vi "智能交通灯.vi"() -> ()   [LabVIEW 2024]
uses:
  <vilib>/Utility/file.llb/Read From Spreadsheet File (DBL).vi
panel:
  in  "?":u16(ring) items=["无", "黄灯常亮", "南北通行", "东西通行"]
  in  "手动\n\n自动":bool
  in  "道路宽度":dbl
  in  "人流量":dbl
  in  "车流量":dbl
  in  "模式切换":bool
  out "日志":string
  out "自动模式":bool
  in  "绿灯时间":i32
  in  "红灯时间":i32
  in  "黄灯时间":i32
  out "手动模式":bool
  out "北红":bool
  out "北绿":bool
  out "北黄":bool
  out "北灯":dbl
  out "南黄":bool
  out "南红":bool
  out "南绿":bool
  out "南灯":dbl
  out "西绿":bool
  out "西黄":bool
  out "西红":bool
  out "西灯":dbl
  out "东黄":bool
  out "东绿":bool
  out "东红":bool
  out "东灯":dbl
  # "交通灯控制交互界面"
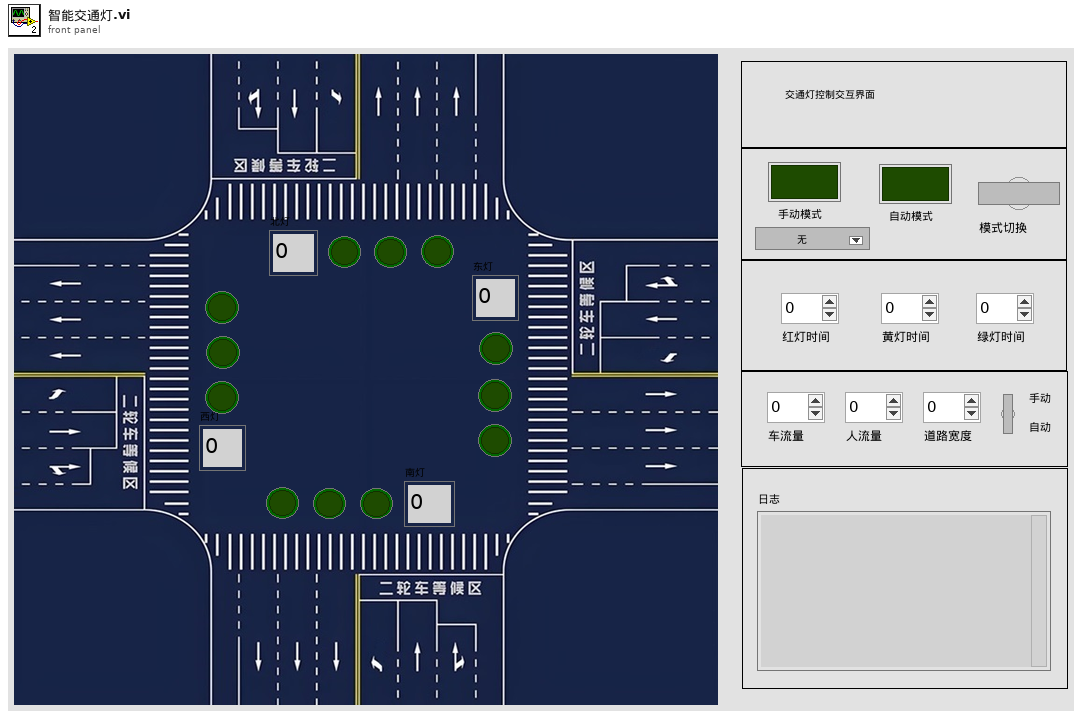
[diagram p1: front panel]
types:
  T1 = cluster{"first row[0]":dbl, "first row[1]":dbl, "first row[2]":dbl}
  T2 = cluster{"[0]":bool, "[1]":bool, "[2]":bool, "[3]":bool, "[4]":bool, "[5]":bool, "[6]":bool, "[7]":bool, "[8]":bool, "[9]":bool, "[10]":bool, "[11]":bool}
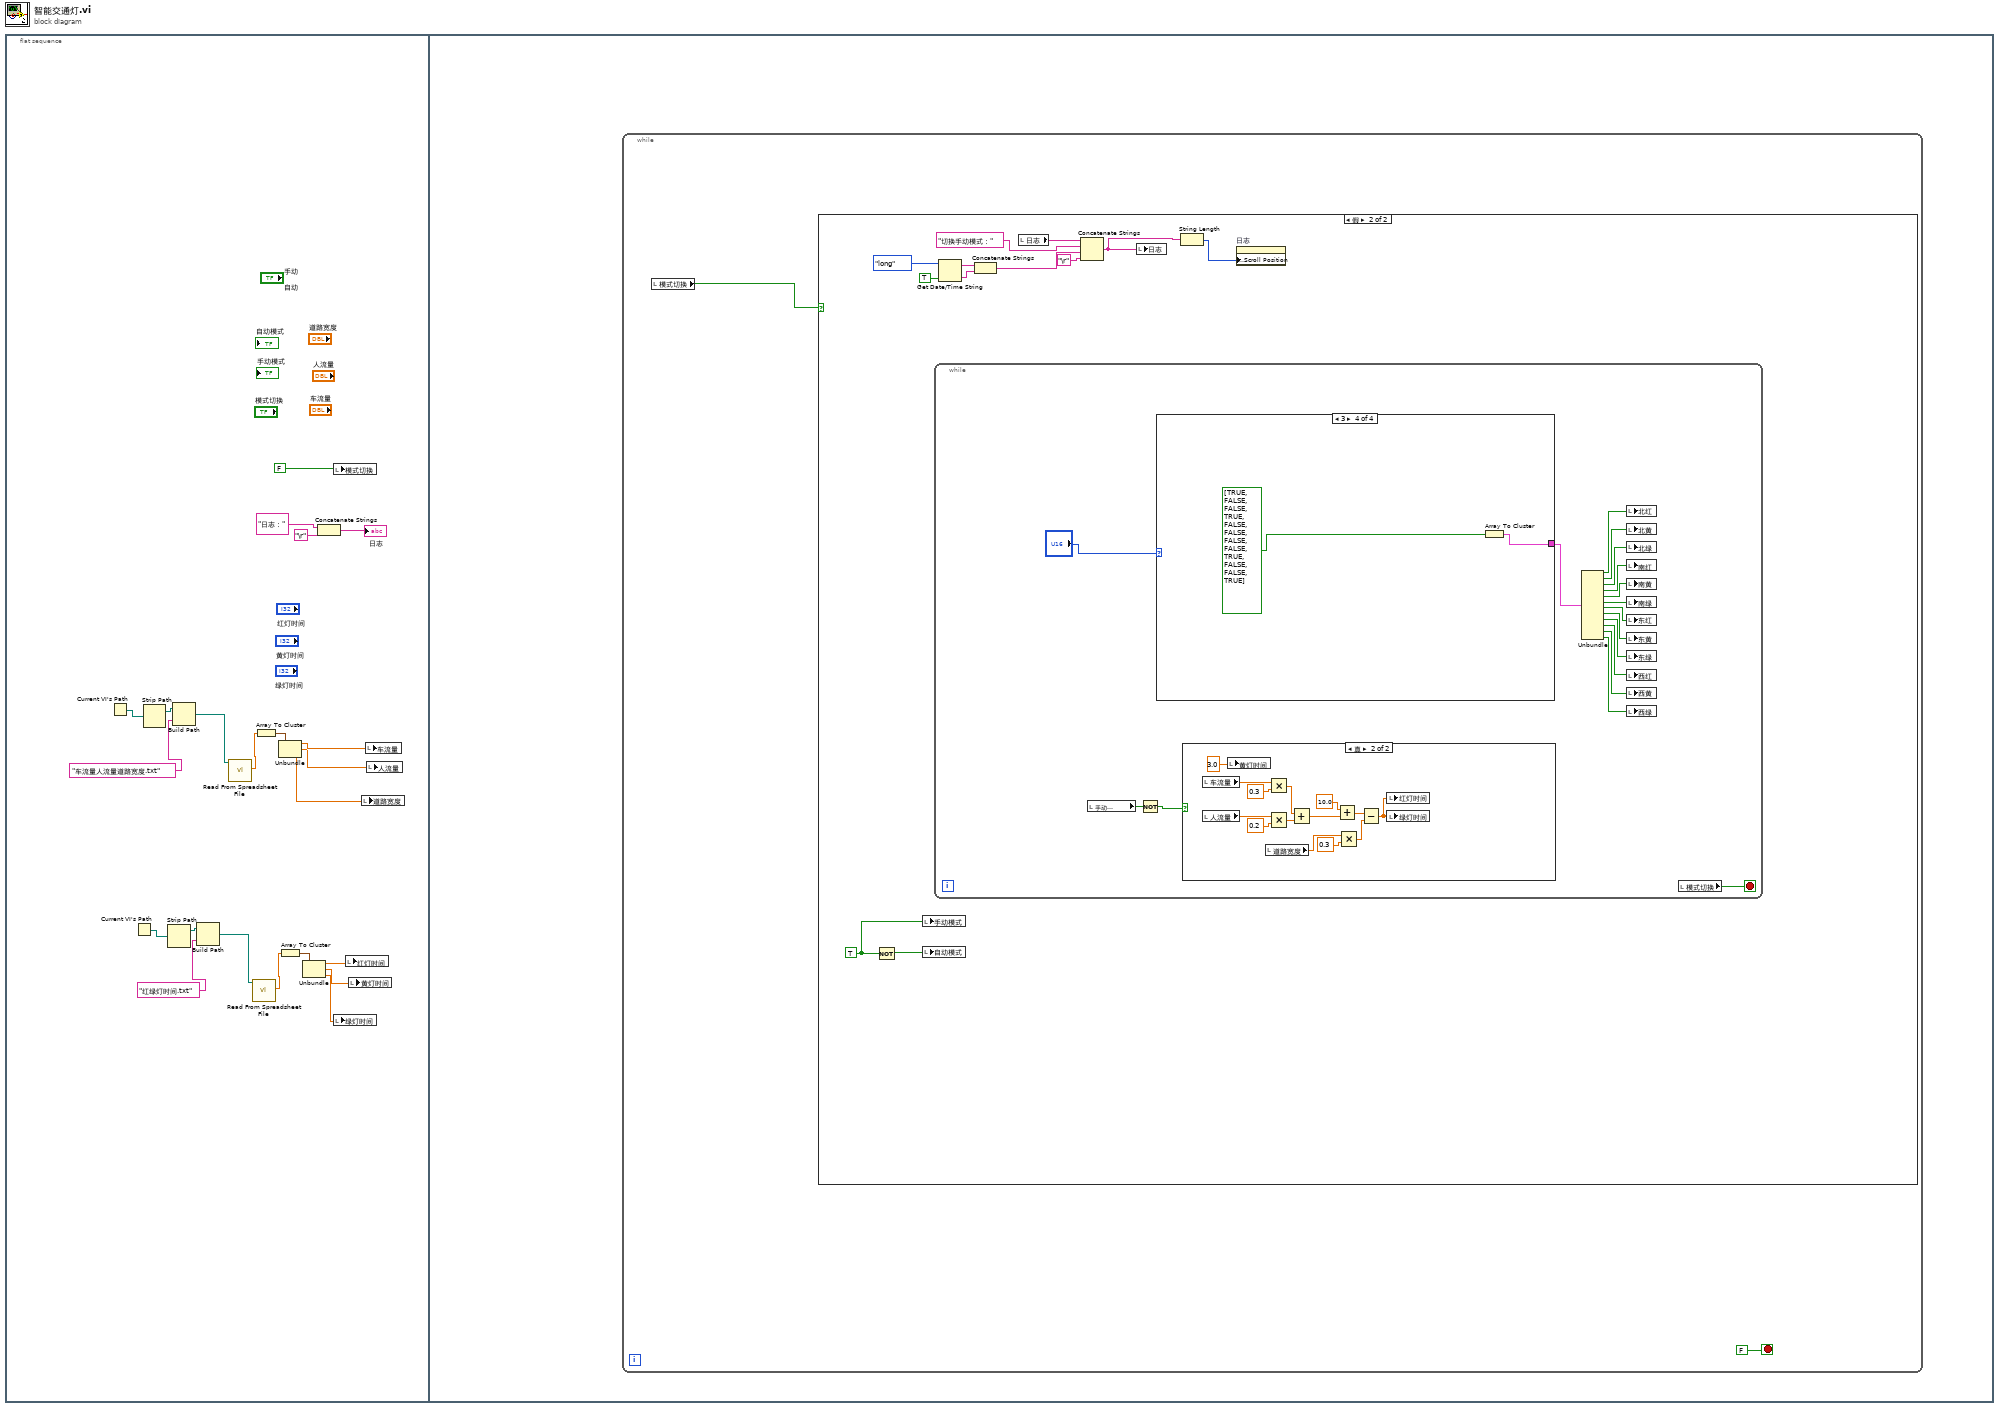
[diagram p0: block diagram]
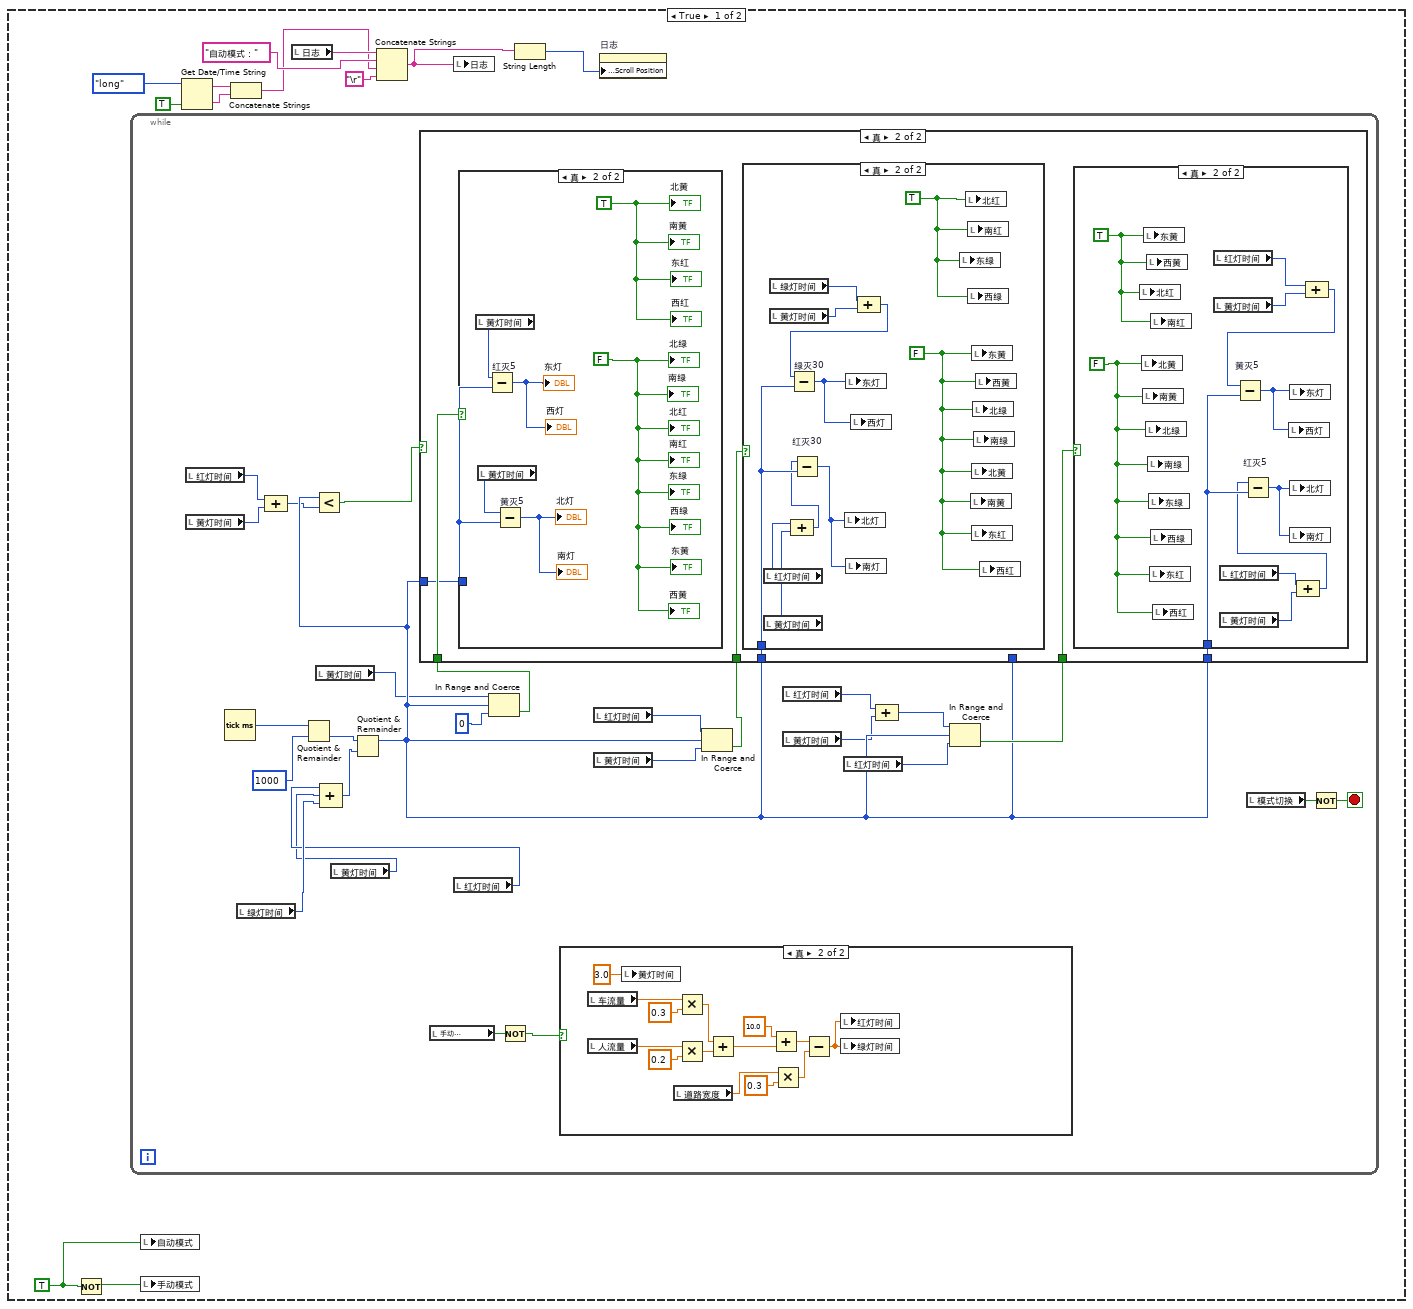
[diagram p2: hidden frame]
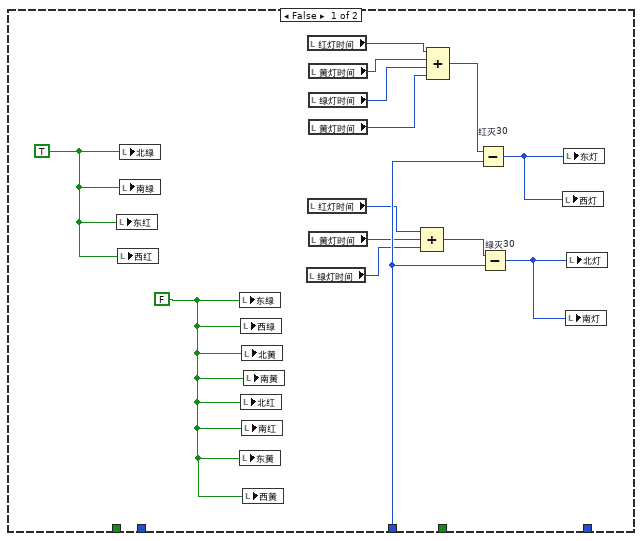
[diagram p4: hidden frame]
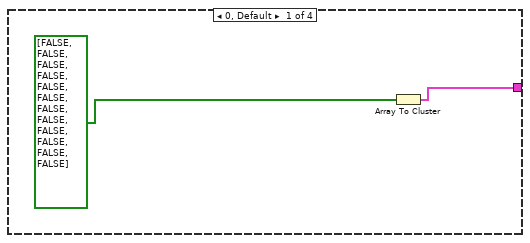
[diagram p8: hidden frame]
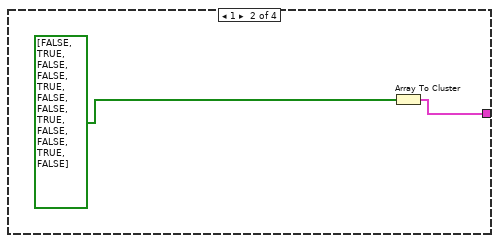
[diagram p9: hidden frame]
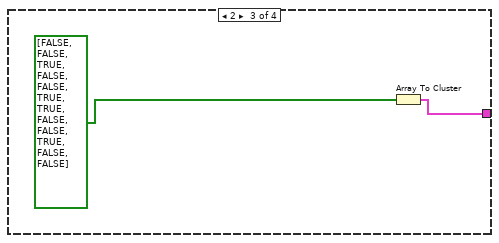
[diagram p10: hidden frame]
diagram:
  n1 = flat-sequence {
    frame #0 {
      n2 = Current VI's Path() -> (path=w4:path)
      n3 = Current VI's Path() -> (path=w18:path)
      n4 = Strip Path(path=w4) -> (stripped path=w5:path)  [unwired: 1 out]
      n5 = Strip Path(path=w18) -> (stripped path=w17:path)  [unwired: 1 out]
      n6 = Build Path(base path=w5, name or relative path="车流量人流量道路宽度.txt" ("名称")) -> (appended path=w7:path)
      n7 = Build Path(base path=w17, name or relative path="红绿灯时间.txt" ("名称")) -> (appended path=w15:path)
      n8 = call-poly <vilib>:"Read From Spreadsheet File.vi"("file path (dialog if empty)"=w7) -> ("first row"=w8:dbl[])  [unwired: 6 in, 4 out]
      n9 = call-poly <vilib>:"Read From Spreadsheet File.vi"("file path (dialog if empty)"=w15) -> ("first row"=w14:dbl[])  [unwired: 6 in, 4 out]
      n10 = Array To Cluster(array=w8) -> (cluster=w9:T1)
      n11 = Unbundle(w9) -> ("first row[0]"=w3:dbl, "first row[1]"=w2:dbl, "first row[2]"=w1:dbl)
      n12 = Array To Cluster(array=w14) -> (cluster=w13:T1)
      n13 = Unbundle(w13) -> ("first row[0]"=w12:dbl, "first row[1]"=w11:dbl, "first row[2]"=w10:dbl)
      n14 = Concatenate Strings("日志：" ("日志"), "\r") -> (→"日志":string)
      n15 = local write "模式切换"(FALSE) -> ()
      n16 = local write "绿灯时间"(w10) -> ()
      n17 = local write "红灯时间"(w12) -> ()
      n18 = local write "黄灯时间"(w11) -> ()
      n19 = local write "道路宽度"(w1) -> ()
      n20 = local write "车流量"(w3) -> ()
      n21 = local write "人流量"(w2) -> ()
    }
    frame #1 {
      n22 = while {
        stop <- FALSE stop-if-true
        n23 = local read "模式切换"() -> (w23:bool)
        n24 = case shown="假" w23 {
          frame True {
            w35 = TRUE
            n25 = Not(x=w35) -> (.not. x?=w36:bool)
            n26 = while {
              stop <- w40 stop-if-true
              n27 = local read "红灯时间"() -> (w51:i32)
              n28 = local read "黄灯时间"() -> (w50:i32)
              n29 = Tick Count (ms)() -> (millisecond timer value=w63:u32)
              n30 = local read "绿灯时间"() -> (w43:i32)
              n31 = Compound Arithmetic op=ADD(w51, w50) -> (w53:i32)
              n32 = Quotient & Remainder(x=w63, y=1000) -> (floor(x/y)=w60:u32)  [unwired: 1 out]
              n33 = local read "黄灯时间"() -> (w49:i32)
              n34 = local read "黄灯时间"() -> (w41:i32)
              n35 = local read "手动\n\n自动"() -> (w38:bool)
              n36 = local read "红灯时间"() -> (w42:i32)
              n37 = Compound Arithmetic op=ADD(w42, w41, w43) -> (w54:i32)
              n38 = Quotient & Remainder(x=w60, y=w54) -> (x-y*floor(x/y)=w55:u32)  [unwired: 1 out]
              n39 = Less?(x=w55, y=w53) -> (x < y?=w59:bool)
              n40 = In Range and Coerce(upper limit=w49, x=w55, lower limit=0) -> (In Range?=w58:bool)  [unwired: 1 out]
              n41 = Not(x=w38) -> (.not. x?=w37:bool)
              n42 = case shown="真" w37 {
                frame False {
                }
                frame True {
                  n43 = local read "车流量"() -> (w77:dbl)
                  n44 = local read "人流量"() -> (w75:dbl)
                  n45 = local write "黄灯时间"(3.0 ("黄灯时间")) -> ()
                  n46 = local read "道路宽度"() -> (w68:dbl)
                  n47 = Multiply(x=w77, y=0.3) -> (x*y=w73:dbl)
                  n48 = Multiply(x=w75, y=0.2) -> (x*y=w72:dbl)
                  n49 = Add(x=w73, y=w72) -> (x+y=w70:dbl)
                  n50 = Add(x=10.0, y=w70) -> (x+y=w69:dbl)
                  n51 = Multiply(x=w68, y=0.3) -> (x*y=w66:dbl)
                  n52 = Subtract(x=w69, y=w66) -> (x-y=w65:dbl)
                  n53 = local write "红灯时间"(w65) -> ()
                  n54 = local write "绿灯时间"(w65) -> ()
                }
              }
              n55 = local read "红灯时间"() -> (w48:i32)
              n56 = local read "黄灯时间"() -> (w47:i32)
              n57 = In Range and Coerce(upper limit=w48, x=w55, lower limit=w47) -> (In Range?=w57:bool)  [unwired: 1 out]
              n58 = local read "红灯时间"() -> (w46:i32)
              n59 = local read "黄灯时间"() -> (w45:i32)
              n60 = local read "红灯时间"() -> (w44:i32)
              n61 = Compound Arithmetic op=ADD(w46, w45) -> (w52:i32)
              n62 = In Range and Coerce(upper limit=w52, x=w55, lower limit=w44) -> (In Range?=w56:bool)  [unwired: 1 out]
              n63 = case shown="真" w59 {
                tunnel: w58 -> [_ w97]
                tunnel: w55 -> [_ w96]
                tunnel: w55 -> [_ w95]
                tunnel: w55 -> [_ w94]
                tunnel: w57 -> [_ w93]
                tunnel: w56 -> [_ w92]
                tunnel: w55 -> [w91 _]
                frame False {
                  w87 = FALSE
                  w88 = TRUE
                  n64 = local write "东红"(w88) -> ()
                  n65 = local write "西红"(w88) -> ()
                  n66 = local write "北绿"(w88) -> ()
                  n67 = local write "南绿"(w88) -> ()
                  n68 = local write "东绿"(w87) -> ()
                  n69 = local write "东黄"(w87) -> ()
                  n70 = local write "西绿"(w87) -> ()
                  n71 = local write "北红"(w87) -> ()
                  n72 = local write "北黄"(w87) -> ()
                  n73 = local write "南红"(w87) -> ()
                  n74 = local write "西黄"(w87) -> ()
                  n75 = local write "南黄"(w87) -> ()
                  n76 = local read "绿灯时间"() -> (w83:i32)
                  n77 = local read "红灯时间"() -> (w81:i32)
                  n78 = local read "红灯时间"() -> (w84:i32)
                  n79 = local read "黄灯时间"() -> (w80:i32)
                  n80 = local read "绿灯时间"() -> (w79:i32)
                  n81 = local read "黄灯时间"() -> (w78:i32)
                  n82 = local read "黄灯时间"() -> (w82:i32)
                  n83 = Compound Arithmetic op=ADD(w84, w82, w83) -> (w86:i32)
                  n84 = Compound Arithmetic op=ADD(w81, w80, w79, w78) -> (w85:i32)
                  n85 = Subtract "红灭30"(x=w85, y=w91) -> (x-y=w90:u32)
                  n86 = Subtract "绿灭30"(x=w86, y=w91) -> (x-y=w89:u32)
                  n87 = local write "西灯"(w90) -> ()
                  n88 = local write "东灯"(w90) -> ()
                  n89 = local write "南灯"(w89) -> ()
                  n90 = local write "北灯"(w89) -> ()
                }
                frame True {
                  n91 = case shown="真" w97 {
                    tunnel: w96 -> [_ w104]
                    frame False {
                    }
                    frame True {
                      w100 = FALSE
                      w103 = TRUE ("布尔")
                      n92 = local read "黄灯时间"() -> (w99:i32)
                      n93 = local read "黄灯时间"() -> (w98:i32)
                      n94 = Subtract "红灭5"(x=w99, y=w104) -> (x-y=→"东灯" →"西灯":u32)
                      n95 = Subtract "黄灭5"(x=w98, y=w104) -> (x-y=→"北灯" →"南灯":u32)
                      "北黄" <- w103
                      "北绿" <- w100
                      "东红" <- w103
                      "东黄" <- w100
                      "北红" <- w100
                      "东绿" <- w100
                      "南黄" <- w103
                      "西红" <- w103
                      "南绿" <- w100
                      "南红" <- w100
                      "西绿" <- w100
                      "西黄" <- w100
                    }
                  }
                  n96 = case shown="真" w93 {
                    tunnel: w94 -> [_ w126]
                    frame False {
                    }
                    frame True {
                      w122 = FALSE
                      w125 = TRUE
                      n97 = local read "红灯时间"() -> (w120:i32)
                      n98 = local read "黄灯时间"() -> (w119:i32)
                      n99 = local read "绿灯时间"() -> (w118:i32)
                      n100 = local read "黄灯时间"() -> (w117:i32)
                      n101 = Compound Arithmetic op=ADD(w120, w119) -> (w121:i32)
                      n102 = Subtract "红灭30"(x=w121, y=w126) -> (x-y=w123:u32)
                      n103 = local write "北灯"(w123) -> ()
                      n104 = local write "南灯"(w123) -> ()
                      n105 = Compound Arithmetic op=ADD(w118, w117) -> (w116:i32)
                      n106 = Subtract "绿灭30"(x=w116, y=w126) -> (x-y=w124:u32)
                      n107 = local write "东灯"(w124) -> ()
                      n108 = local write "西灯"(w124) -> ()
                      n109 = local write "东绿"(w125) -> ()
                      n110 = local write "北红"(w125) -> ()
                      n111 = local write "南红"(w125) -> ()
                      n112 = local write "西绿"(w125) -> ()
                      n113 = local write "南黄"(w122) -> ()
                      n114 = local write "东黄"(w122) -> ()
                      n115 = local write "北黄"(w122) -> ()
                      n116 = local write "东红"(w122) -> ()
                      n117 = local write "北绿"(w122) -> ()
                      n118 = local write "南绿"(w122) -> ()
                      n119 = local write "西黄"(w122) -> ()
                      n120 = local write "西红"(w122) -> ()
                    }
                  }
                  n121 = case shown="真" w92 {
                    tunnel: w95 -> [_ w115]
                    frame False {
                    }
                    frame True {
                      w113 = FALSE
                      w114 = TRUE
                      n122 = local write "北红"(w114) -> ()
                      n123 = local write "北黄"(w113) -> ()
                      n124 = local write "南黄"(w113) -> ()
                      n125 = local write "东黄"(w114) -> ()
                      n126 = local write "北绿"(w113) -> ()
                      n127 = local write "西黄"(w114) -> ()
                      n128 = local write "南绿"(w113) -> ()
                      n129 = local write "东绿"(w113) -> ()
                      n130 = local write "东红"(w113) -> ()
                      n131 = local write "南红"(w114) -> ()
                      n132 = local write "西绿"(w113) -> ()
                      n133 = local write "西红"(w113) -> ()
                      n134 = local read "红灯时间"() -> (w105:i32)
                      n135 = local read "黄灯时间"() -> (w106:i32)
                      n136 = local read "红灯时间"() -> (w108:i32)
                      n137 = local read "黄灯时间"() -> (w107:i32)
                      n138 = Compound Arithmetic op=ADD(w108, w107) -> (w109:i32)
                      n139 = Subtract "红灭5"(x=w109, y=w115) -> (x-y=w112:u32)
                      n140 = local write "北灯"(w112) -> ()
                      n141 = local write "南灯"(w112) -> ()
                      n142 = Compound Arithmetic op=ADD(w105, w106) -> (w110:i32)
                      n143 = Subtract "黄灭5"(x=w110, y=w115) -> (x-y=w111:u32)
                      n144 = local write "西灯"(w111) -> ()
                      n145 = local write "东灯"(w111) -> ()
                    }
                  }
                }
              }
              n146 = local read "模式切换"() -> (w39:bool)
              n147 = Not(x=w39) -> (.not. x?=w40:bool)
            }
            n148 = local write "自动模式"(w35) -> ()
            n149 = local write "手动模式"(w36) -> ()
            n150 = Get Date/Time String(date format (0)=enum16{"short", "long", "abbreviated"}."long" ("日期格式(0)"), want seconds? (F)=TRUE ("需要秒？(F)")) -> (date string=w28:string, time string=w29:string)  [unwired: 1 in]
            n151 = Concatenate Strings(w28, w29) -> (w26:string)
            n152 = local read "日志"() -> (w27:string)
            n153 = Concatenate Strings(w27, "自动模式：" ("日志"), w26, "\r") -> (w34:string)
            n154 = local write "日志"(w34) -> ()
            n155 = String Length(string=w34) -> (length=w25:i32)
            n156 = property on="日志" class="Str"("Text.Scroll Position"=w25) -> ()  [unwired: 2 in, 2 out]
          }
          frame False {
            w127 = TRUE
            n157 = Not(x=w127) -> (.not. x?=w128:bool)
            n158 = local write "手动模式"(w127) -> ()
            n159 = local write "自动模式"(w128) -> ()
            n160 = while {
              stop <- w155 stop-if-true
              n161 = local read "手动\n\n自动"() -> (w154:bool)
              n162 = Not(x=w154) -> (.not. x?=w153:bool)
              n163 = case shown="3" "?" {
                tunnel: [w157 w158 w160 w162] -> w151
                frame 0, Default {
                  n164 = Array To Cluster(array=bool[] [FALSE, FALSE, FALSE, FALSE, FALSE, FALSE, FALSE, FALSE, FALSE, FALSE, FALSE, FALSE]) -> (cluster=w157:T2)
                }
                frame 1 {
                  n165 = Array To Cluster(array=bool[] [FALSE, TRUE, FALSE, FALSE, TRUE, FALSE, FALSE, TRUE, FALSE, FALSE, TRUE, FALSE]) -> (cluster=w158:T2)
                }
                frame 2 {
                  n166 = Array To Cluster(array=bool[] [FALSE, FALSE, TRUE, FALSE, FALSE, TRUE, TRUE, FALSE, FALSE, TRUE, FALSE, FALSE]) -> (cluster=w160:T2)
                }
                frame 3 {
                  n167 = Array To Cluster(array=bool[] [TRUE, FALSE, FALSE, TRUE, FALSE, FALSE, FALSE, FALSE, TRUE, FALSE, FALSE, TRUE]) -> (cluster=w162:T2)
                }
              }
              n168 = case shown="真" w153 {
                frame False {
                }
                frame True {
                  n169 = local read "车流量"() -> (w177:dbl)
                  n170 = local read "人流量"() -> (w175:dbl)
                  n171 = local write "黄灯时间"(3.0 ("黄灯时间")) -> ()
                  n172 = local read "道路宽度"() -> (w168:dbl)
                  n173 = Multiply(x=w177, y=0.3) -> (x*y=w173:dbl)
                  n174 = Multiply(x=w175, y=0.2) -> (x*y=w172:dbl)
                  n175 = Add(x=w173, y=w172) -> (x+y=w170:dbl)
                  n176 = Add(x=10.0, y=w170) -> (x+y=w169:dbl)
                  n177 = Multiply(x=w168, y=0.3) -> (x*y=w166:dbl)
                  n178 = Subtract(x=w169, y=w166) -> (x-y=w165:dbl)
                  n179 = local write "红灯时间"(w165) -> ()
                  n180 = local write "绿灯时间"(w165) -> ()
                }
              }
              n181 = Unbundle(w151) -> ("[0]"=w150:bool, "[1]"=w149:bool, "[2]"=w148:bool, "[3]"=w147:bool, "[4]"=w146:bool, "[5]"=w145:bool, "[6]"=w144:bool, "[7]"=w143:bool, "[8]"=w142:bool, "[9]"=w141:bool, "[10]"=w140:bool, "[11]"=w139:bool)
              n182 = local write "北红"(w150) -> ()
              n183 = local write "北黄"(w149) -> ()
              n184 = local write "北绿"(w148) -> ()
              n185 = local write "南红"(w147) -> ()
              n186 = local write "南黄"(w146) -> ()
              n187 = local write "南绿"(w145) -> ()
              n188 = local write "东红"(w144) -> ()
              n189 = local write "东黄"(w143) -> ()
              n190 = local write "东绿"(w142) -> ()
              n191 = local write "西红"(w141) -> ()
              n192 = local write "西黄"(w140) -> ()
              n193 = local write "西绿"(w139) -> ()
              n194 = local read "模式切换"() -> (w155:bool)
            }
            n195 = Get Date/Time String(date format (0)=enum16{"short", "long", "abbreviated"}."long" ("日期格式(0)"), want seconds? (F)=TRUE ("需要秒？(F)")) -> (date string=w134:string, time string=w135:string)  [unwired: 1 in]
            n196 = Concatenate Strings(w134, w135) -> (w137:string)
            n197 = local read "日志"() -> (w131:string)
            n198 = Concatenate Strings(w131, "切换手动模式：" ("日志"), w137, "\r") -> (w138:string)
            n199 = local write "日志"(w138) -> ()
            n200 = String Length(string=w138) -> (length=w129:i32)
            n201 = property on="日志" class="Str"("Text.Scroll Position"=w129) -> ()  [unwired: 2 in, 2 out]
          }
        }
      }
    }
  }
